vi "feet to encoder ticks.vi"(11 "Distance in feet wanted":dbl) -> (3 "Encoder Ticks":dbl)   [LabVIEW 2017]
panel:
  # "Dosen't do anything right now"
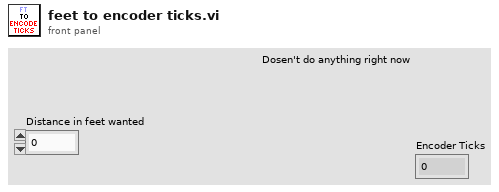
[diagram p1: front panel]
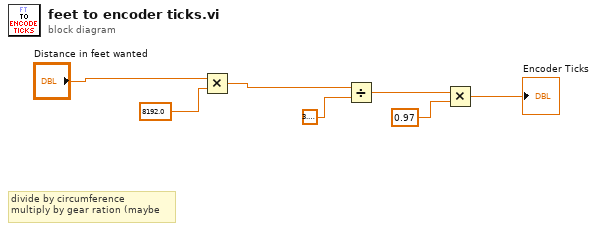
[diagram p0: block diagram]
diagram:
  # "divide by circumference\nmultiply by gear ration (maybe"
  n1 = Multiply(x="Distance in feet wanted", y=8192.0) -> (x*y=w4:dbl)
  n2 = Divide(x=w4, y=3.141592653589793) -> (x/y=w3:dbl)
  n3 = Multiply(x=w3, y=0.97) -> (x*y=→"Encoder Ticks":dbl)
